vi "Quest Enable Register.vi"(8 "error in (no error)":errorcluster, 9 "Register Bit(0)":i32 min=0 max=255 step=1, 10 "Channel Select":enum16{"Channel 1", "Channel 2", "Channel 3"}(ring), 11 "Visa Resource Name IN":refnum<visa-resource-name>) -> (0 "error out":errorcluster, 3 "Visa Resource Name OUT":refnum<visa-resource-name>)   [LabVIEW 2018, in "Keithley KE22xx Series.lvlib"]
doc: "To modify Quest Enable Register for specified channel."
uses:
  Keithley KE22xx Series.lvlib
panel:
  # "© 2012 Keithley Instruments, Inc. ALL RIGHTS RESERVED"
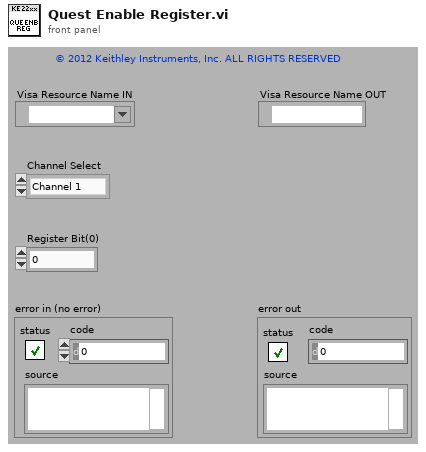
[diagram p1: front panel]
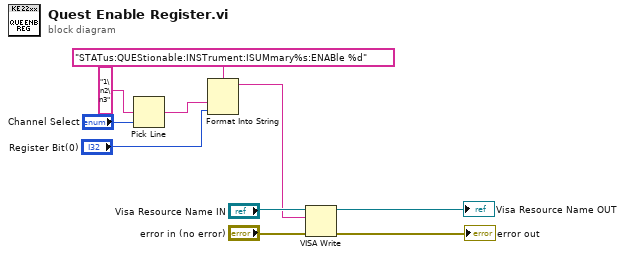
[diagram p0: block diagram]
diagram:
  n1 = Pick Line(multi-line string="1\n2\n3", line index="Channel Select") -> (output string=w5:string)  [unwired: 1 in]
  n2 = Format Into String(format string="STATus:QUEStionable:INSTrument:ISUMmary%s:ENABle %d", w5, "Register Bit(0)") -> (resulting string=w4:string)  [unwired: 2 in, 1 out]
  n3 = VISA Write(VISA resource name="Visa Resource Name IN", write buffer=w4, error in (no error)="error in (no error)") -> (VISA resource name out=→"Visa Resource Name OUT":refnum<visa-resource-name>, error out=→"error out":errorcluster)  [unwired: 1 out]
